vi "Read Msg Input.vi"(10 "Msg Input":refnum<class "Msg Input.lvclass">) -> (4 "Teller":T1 {"Time" format="%<%x %.3X>T"})   [LabVIEW 2020, in "jettl.lvlib" / "Start jettl Msg.lvlib" / "Start Msg Input.lvlib"]
doc: "jettl 6.14.1.98\nNathan Davis - Nathan Davis\nCopyright (c) 2026, Nathan Davis\nMIT"
uses:
  Start Msg Input.lvlib
  Msg Input/Msg Input.lvclass
  Start Msg Input/Start Msg Input.lvclass
  Relation.ctl
  jettl.lvlib
  Teller Metadata/Teller Metadata.lvclass
  Teller.ctl
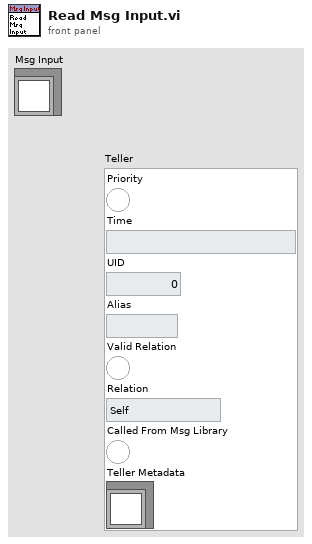
[diagram p1: front panel]
types:
  T1 = typedef "jettl.lvlib/Teller.ctl" = cluster{"Priority":bool, "Time":timestamp, "UID":i32, "Alias":string, "Valid Relation":bool, "Relation":T2, "Called From Msg Library":bool, "Teller Metadata":refnum<class "Teller Metadata.lvclass">}
  T2 = typedef "jettl.lvlib/Relation.ctl" = enum16{"Self", "Parent", "Child"}
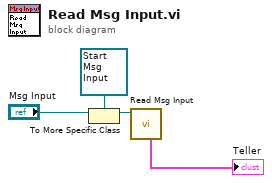
[diagram p0: block diagram]
diagram:
  n1 = To More Specific Class(target class=refnum<class "Start Msg Input.lvclass"> refnum ("_Template.lvlib:Templates.lvlib:TEMPLATE Msg.lvlib:TEMPLATE Msg Input.lvlib:TEMPLATE Msg Input.lvclass"), reference="Msg Input") -> (specific class reference=w3:refnum<class "Start Msg Input.lvclass">)  [unwired: 1 in, 1 out]
  n2 = call "Read Msg Input.vi"("Start Msg Input in"=w3) -> ("Teller"=→"Teller":T1)  [unwired: 10 in]
